vi "CropAndCombineAndShiftTIFFs_list.vi"() -> ()   [LabVIEW 2011]
uses:
  Library/tiff/TiffModules/AddTiffPage_U16_text_res.vi
panel:
  in  "Clear string":bool=TRUE
  out "Frame":i32
  in  "in y":bool
  in  "Shiftloop":i32
  in  "Shift per frame":dbl=2.9
  in  "BigTiff,Endian":u16(ring)=257 items=["Big-Endian"=0, "Native"=1, "Little-Endian"=2, "BigTiff-Big-Endian"=256, "Bigtiff,Native"=257, "Biftiff,Littleendian"=258]
  in  "Stop at offset:":u64=429496729500
  out "Input-File":i32
  out "AfterDIRoffset":u64 format="%09d"
  in  "Files":path[](array[path])
  in  "y-length":i32=1040
  in  "y-start":i32
  in  "x-length":i32=2286
  in  "x-start":i32
  out "Input-page":i32
  out "string":string
  in  "xy-resolution":cluster{"x":dbl, "y":dbl}={"x"=1.0, "y"=1.0}
  out "Out":u16[][](graph)
  out "In":u16[][](graph)
  # "select all tiff files, with correct order!\nenter crop data (wie IJ!)\nrun\nnew name first with _cropcombine.tif\nstops at max tiff-offset 2^32"
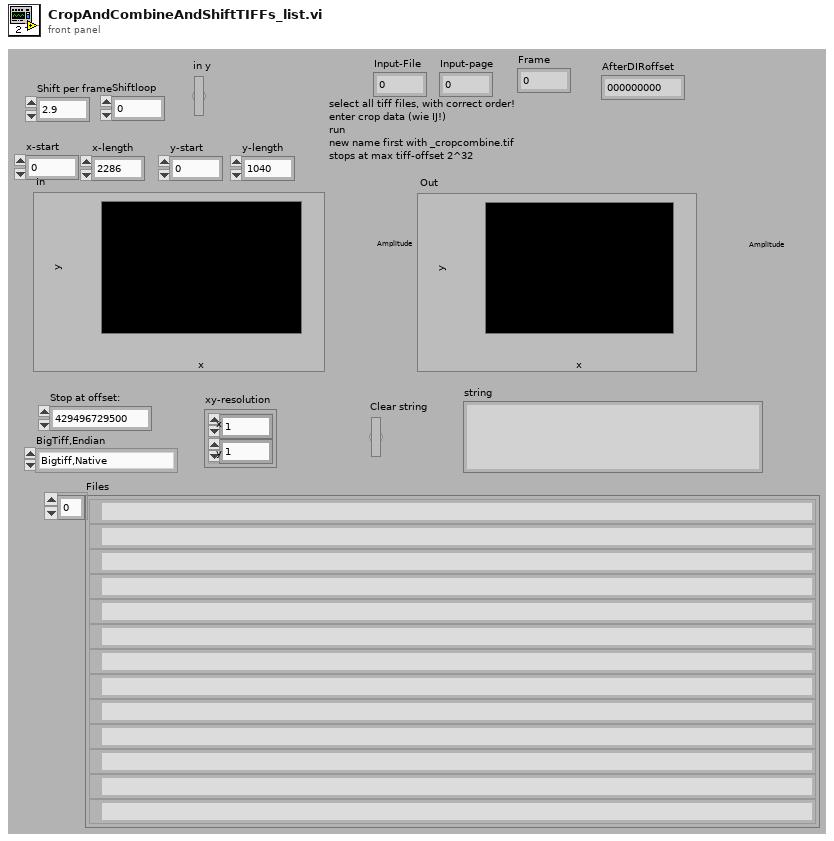
[diagram p1: front panel]
types:
  T1 = cluster{"Tiff refnum":refnum<file>, "BigTiff,Endian":u16}
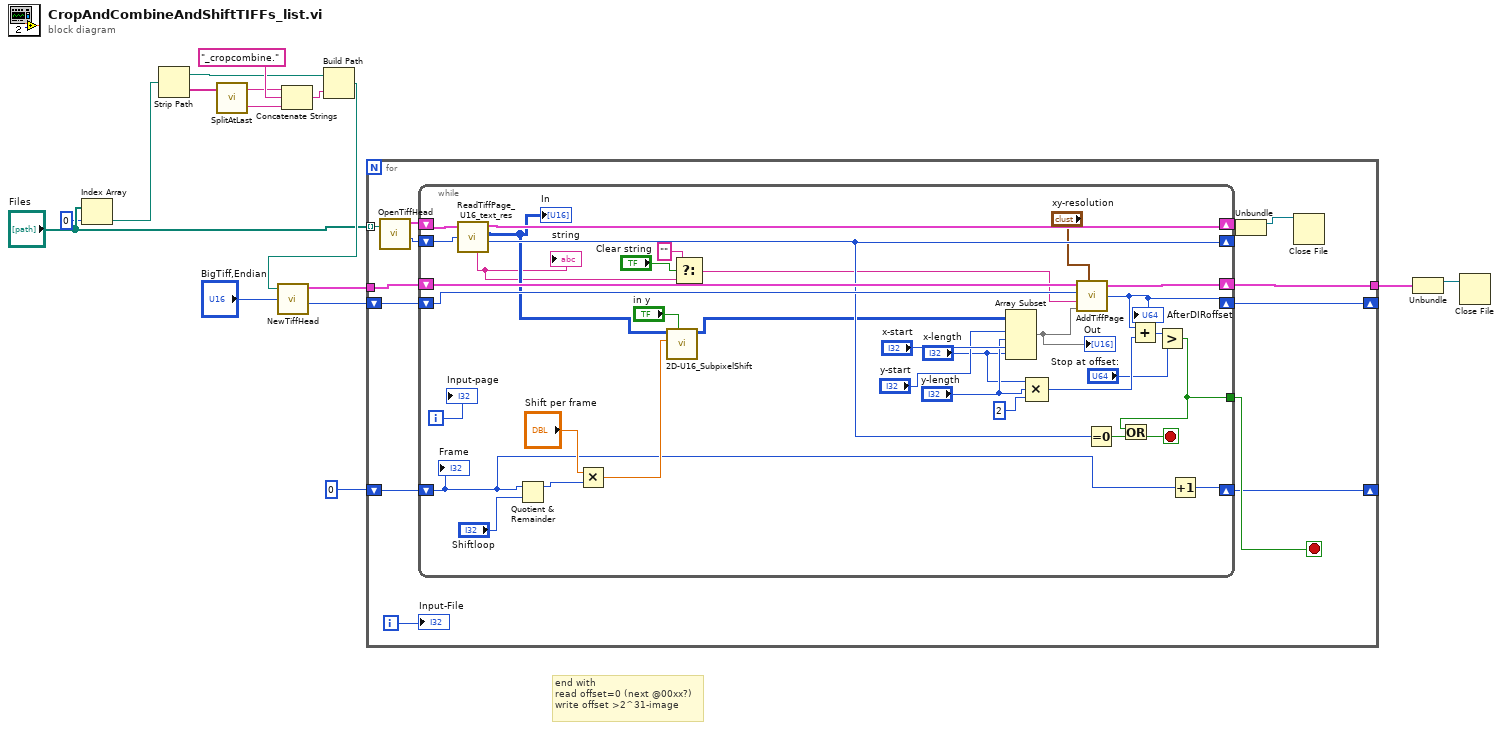
[diagram p0: block diagram]
diagram:
  # "end with \nread offset=0 (next @00xx?)\nwrite offset >2^31-image"
  n1 = Index Array(array="Files", index=0) -> (element=w3:path)
  n2 = Strip Path(path=w3) -> (stripped path=w6:path, name=w7:string)
  n3 = call "SplitAtLast.vi"("In-String"=w7) -> ("end"=w15:string, "Front (default)"=w8:string)  [unwired: 1 in]
  n4 = Concatenate Strings(w8, "_cropcombine." ("String"), w15) -> (w14:string)
  n5 = Build Path(base path=w6, name or relative path=w14) -> (appended path=w13:path)
  n6 = call "NewTiffHead.vi"("file path"=w13, "BigTiff,Endian"="BigTiff,Endian") -> ("TIFF file"=w12:T1, "Place for first IFD (8,eof-position)"=w11:u64)  [unwired: 2 in, 1 out]
  n7 = for {
    tunnel: w12 -> [w28]
    tunnel: [w24] -> w10
    tunnel: "Files" -> [w22] mode=indexing
    shift-right: [w19] -> _
    shift-left: w11 -> [w26]
    shift-right: [w17] -> _
    shift-left: 0 -> [w18]
    i -> [w20]
    stop <- w21 stop-if-true
    n8 = call "OpenTiffHead.vi"("file path"=w22) -> ("TIFF file"=w29:T1, "first Diroffset"=w27:u64)  [unwired: 2 in, 1 out]
    n9 = while {
      shift-right: [w56] -> w25
      shift-left: w29 -> [w58]
      shift-right: [w63] -> w24
      shift-left: w28 -> [w64]
      shift-right: [w55] -> _
      shift-left: w27 -> [w57]
      shift-right: [w49] -> w19
      shift-left: w26 -> [w62]
      tunnel: [w44] -> w21
      shift-right: [w40] -> w17
      shift-left: w18 -> [w35]
      i -> [w60]
      stop <- w45 stop-if-true
      n10 = call "ReadTiffPage_U16_text_res.vi"("TIFF file"=w58, "IFDoffset"=w57) -> ("TIFF file out"=w56:T1, "16-bit pixmap"=w43:u16[][], "string"=w32:string, "Next offset"=w55:i64)  [unwired: 3 in, 2 out]
      "In" <- w43
      "string" <- w32
      n11 = Quotient & Remainder(x=w35, y="Shiftloop") -> (x-y*floor(x/y)=w38:i32)  [unwired: 1 out]
      n12 = Multiply(x="Shift per frame", y=w38) -> (x*y=w36:dbl)
      n13 = call "2D-U16_SubpixelShift.vi"("Shift in y"="in y", "Shift"=w36, "U16-Array"=w43) -> ("U16-Array result"=w42:u16[][])  [unwired: 8 in]
      n14 = Select(t="", s="Clear string", f=w32) -> (s? t:f=w33:string)
      n15 = Array Subset(array=w42, index (row)="y-start", length (row)="y-length", index (col)="x-start", length (col)="x-length") -> (w59:u16[][])
      "Out" <- w59
      n16 = Compound Arithmetic op=MULTIPLY("x-length", "y-length", u64 2 ("value")) -> (w48:u64)
      n17 = call-poly "AddTiffPage.vi"("TIFF file"=w64, "After last DIROffset"=w62, "Text"=w33, "16-bit pixmap x, y"=w59, "Pixelsize [µm]"="xy-resolution") -> ("TIFF file"=w63:T1, "AfterDIRoffset"=w49:u64)  [unwired: 1 out]
      "AfterDIRoffset" <- w49
      n18 = Equal To 0?(x=w55) -> (x = 0?=w61:bool)
      n19 = Add(x=w49, y=w48) -> (x+y=w47:u64)
      n20 = Greater?(x=w47, y="Stop at offset:") -> (0:w44:bool)
      n21 = Or(x=w44, y=w61) -> (x .or. y?=w45:bool)
      n22 = Increment(x=w35) -> (x+1=w40:i32)
      "Input-page" <- w60
      "Frame" <- w35
    }
    n23 = Unbundle(w25) -> ("Tiff refnum"=w23:refnum<file>)  [unwired: 1 out]
    n24 = Close File(refnum=w23) -> ()  [unwired: 1 in, 2 out]
    "Input-File" <- w20
  }
  n25 = Unbundle(w10) -> ("Tiff refnum"=w9:refnum<file>)  [unwired: 1 out]
  n26 = Close File(refnum=w9) -> ()  [unwired: 1 in, 2 out]
